vi "FTW-JSON-Format-Pair.vi"(1 "Prepend to Pair":string="\n  ", 2 "Value":string, 3 "Key":string) -> (0 "JSON Pair":string)   [LabVIEW 2012]
panel:
  # "Inputs"
  # "Outputs"
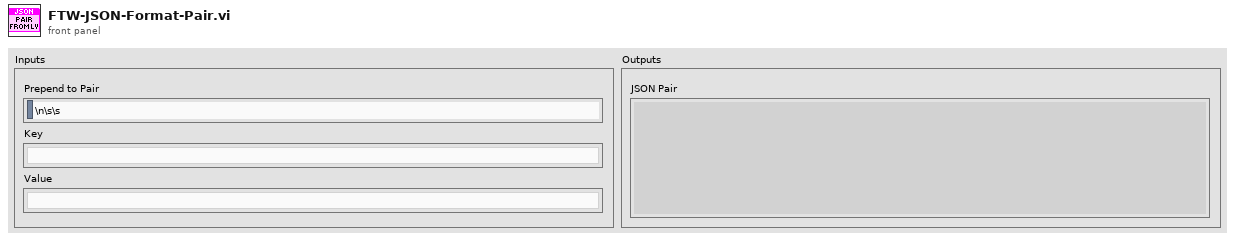
[diagram p1: front panel]
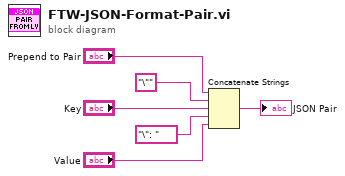
[diagram p0: block diagram]
diagram:
  n1 = Concatenate Strings("Prepend to Pair", "\"" ("String to Repeat"), "Key", "\": " ("String to Repeat"), "Value") -> (→"JSON Pair":string)
